vi "test.vi"() -> ()   [LabVIEW 2017]
uses:
  <vilib>/NIfbLib/NIFBDevice.llb/FF Device Create Block(AI).vi
  <vilib>/NIfbLib/NIFBDevice.llb/FF Device Create Block(AO).vi
panel:
  out "error out":errorcluster
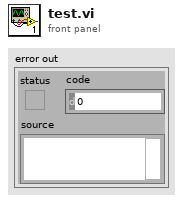
[diagram p1: front panel]
types:
  T1 = cluster{"input high":sgl, "input low":sgl, "unit":enum8{"Voltage", "Ampere", "Kelvin", "Celsius", "Ohm", "Percent"}, "decimal":i8}
  T2 = cluster{"input low":sgl, "input high":sgl, "unit":enum8{"Voltage", "Ampere", "Kelvin", "Celsius", "Ohm", "Percent"}, "decimal":i8}
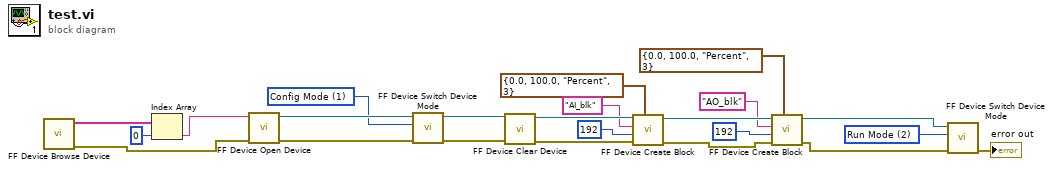
[diagram p0: block diagram]
diagram:
  w4 = u8 2 items=["Config Mode"=1, " Run Mode"=2] ("target mode")
  w17 = u8 1 items=["Config Mode"=1, " Run Mode"=2] ("target mode")
  n1 = call <vilib>:"FF Device Browse Device.vi"() -> ("error out"=w20:errorcluster, "interface names"=w23:string[])  [unwired: 10 in]
  n2 = Index Array(array=w23, index=0) -> (element=w21:string)
  n3 = call <vilib>:"FF Device Open Device.vi"("error in (no error)"=w20, "interface name"=w21) -> ("error out"=w18:errorcluster, "device out"=w19:refnum<k20>)  [unwired: 8 in]
  n4 = call <vilib>:"FF Device Switch Device Mode.vi"("error in (no error)"=w18, "target mode"=w17, "device in"=w19) -> ("error out"=w15:errorcluster, "device out"=w16:refnum<k20>)  [unwired: 7 in]
  n5 = call <vilib>:"FF Device Clear Device.vi"("error in (no error)"=w15, "device in"=w16) -> ("error out"=w13:errorcluster, "device out"=w14:refnum<k20>)  [unwired: 8 in]
  n6 = call-poly <vilib>:"FF Device Create Block.vi"("analog configuration data"=T2 {"input low"=0.0, "input high"=100.0, "unit"=enum."Percent", "decimal"=3}, "error in (no error)"=w13, "execution time (192 ms)"=u32 192 ("execution time (192ms)"), "block ID"="AI_blk", "device in"=w14) -> ("error out"=w5:errorcluster, "device out"=w9:refnum<k20>)  [unwired: 4 in, 1 out]
  n7 = call-poly <vilib>:"FF Device Create Block.vi"("analog configuration data"=T1 {"input high"=0.0, "input low"=100.0, "unit"=enum."Percent", "decimal"=3}, "error in (no error)"=w5, "execution time (192 ms)"=u32 192 ("execution time (192ms)"), "block ID"="AO_blk", "device in"=w9) -> ("error out"=w2:errorcluster, "device out"=w3:refnum<k20>)  [unwired: 4 in, 1 out]
  n8 = call <vilib>:"FF Device Switch Device Mode.vi"("error in (no error)"=w2, "target mode"=w4, "device in"=w3) -> ("error out"=→"error out":errorcluster)  [unwired: 7 in, 1 out]
